vi "globalTearDown.vi"(8 "error in (no error)":errorcluster, 11 "Instrument Addon Host API Tests in":refnum<class "Instrument Addon Host API Tests.lvclass">) -> (0 "error out":errorcluster, 3 "Instrument Addon Host API Tests out":refnum<class "Instrument Addon Host API Tests.lvclass">)   [LabVIEW 2019, in "Instrument Addon Host API Tests.lvclass"]
uses:
  Instrument Addon Host API Tests.lvclass
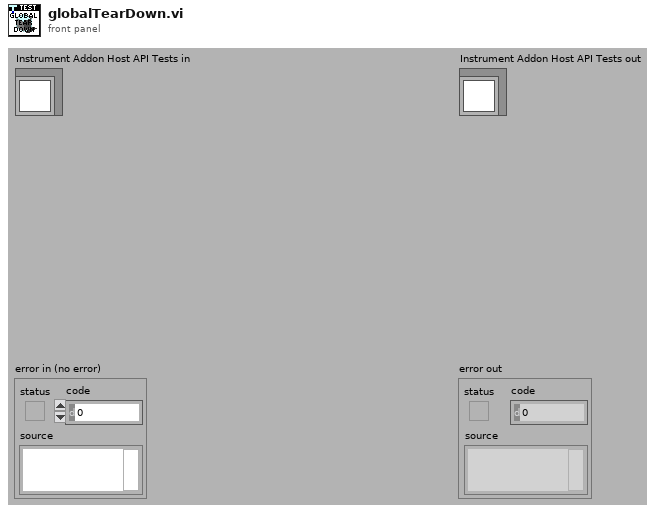
[diagram p1: front panel]
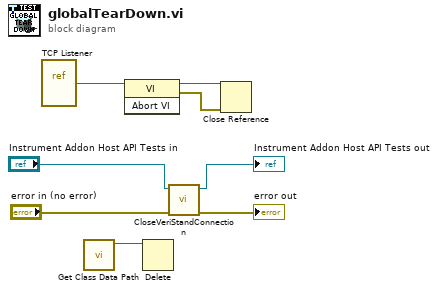
[diagram p0: block diagram]
diagram:
  n1 = vi-ref "TCP Listener.vi"() -> (w8:refnum<vi>)
  n2 = call "Get Class Data Path.vi"() -> ("Class Data File Path"=w5:path)  [unwired: 11 in]
  n3 = invoke class="VI" method="Abort VI"(reference=w8) -> (reference out=w7:refnum<vi>, error out=w6:errorcluster)  [unwired: 2 in, 1 out]
  n4 = Delete(path (use dialog)=w5) -> ()  [unwired: 4 in, 3 out]
  n5 = call-dynamic "CloseVeriStandConnection.vi"("error in (no error)"="error in (no error)", "VeriStand Test Case in"="Instrument Addon Host API Tests in") -> ("error out"=→"error out":errorcluster, "VeriStand Test Case out"=→"Instrument Addon Host API Tests out":refnum<class "Instrument Addon Host API Tests.lvclass">)  [unwired: 8 in]
  n6 = Close Reference(reference=w7, error in (no error)=w6) -> ()  [unwired: 1 out]
